vi "3axis continuous readout.vi"(6 "error in (no error)":errorcluster, 11 "VISA Gaussmeter":refnum<visa-resource-name>="GPIB1::11::INSTR") -> (4 "error out":errorcluster, 5 "VISA resource name":refnum<visa-resource-name>)   [LabVIEW 2013]
uses:
  gaussmeter channels.ctl
panel:
  in  "stop":bool
  in  "sample interval (sec)":dbl=0.1 format="%#_13g"
  out "Channel 3":dbl format="%.2f"
  in  "channel 3":T1=enum."Z"
  out "Channel 3":cluster{dbl, dbl}[](graph)
  in  "channel 2":T1=enum."Y"
  in  "channel 1":T1
  out "Channel 2":cluster{dbl, "magnetic field (T)":dbl}[](graph)
  out "Channel 1":cluster{dbl, dbl}[](graph)
  out "Channel 2":dbl format="%.2f"
  out "Channel 1":dbl format="%.2f"
  # "This .vi reads continuously \nthe values from\nthe Gaussmeter."
  # "Be aware that Hall sensors have\na stabilization time of approx. 3 sec and max. readout rate Gaussmeter: 18 rds/s"
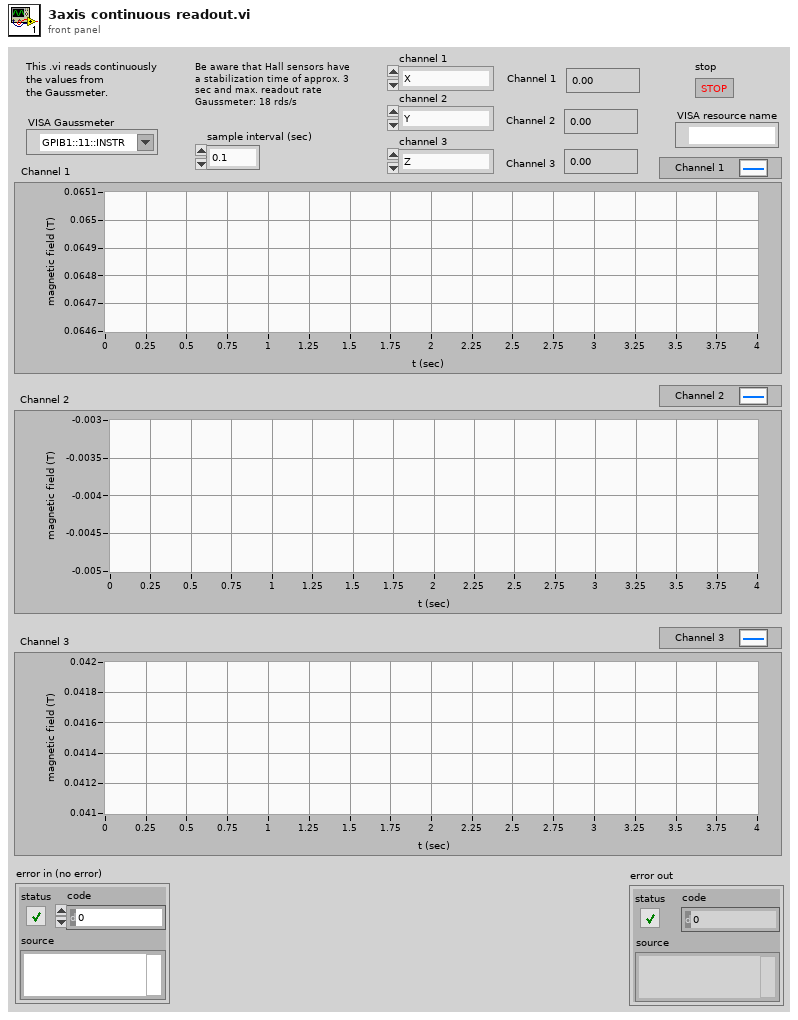
[diagram p1: front panel]
types:
  T1 = typedef "gaussmeter channels.ctl" = enum16{"X", "Y", "Z", "Vec"}
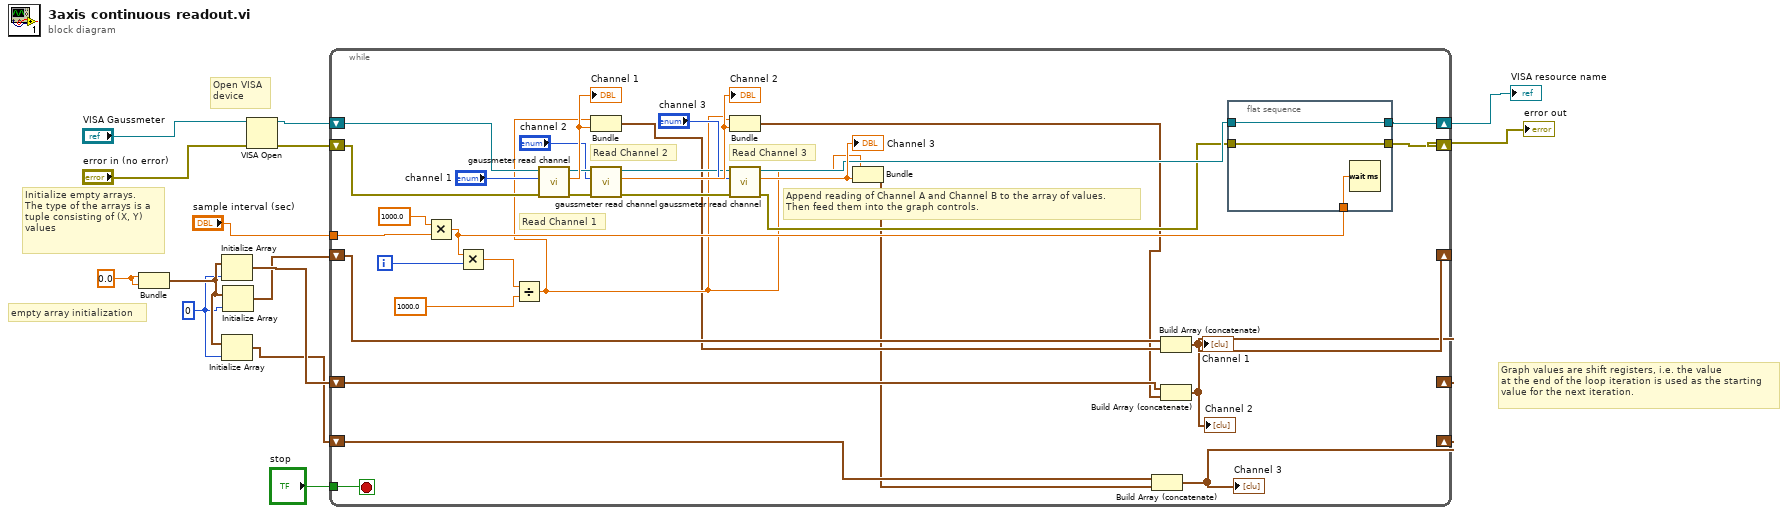
[diagram p0: block diagram]
diagram:
  w4 = 0
  w6 = 0.0
  # "empty array initialization"
  # "Graph values are shift registers, i.e. the value\nat the end of the loop iteration is used as the starting\nvalue for the next iteration."
  # "Initialize empty arrays.\nThe type of the arrays is a tuple consisting of (X, Y) values"
  # "Open VISA\ndevice"
  n1 = Bundle(w6, w6) -> (w5:cluster{dbl, dbl})  [unwired: 1 in]
  n2 = Initialize Array(w5, w4) -> (w10:cluster{dbl, dbl}[])
  n3 = Initialize Array(w5, w4) -> (w3:cluster{dbl, dbl}[])
  n4 = Initialize Array(w5, w4) -> (w9:cluster{dbl, dbl}[])
  n5 = VISA Open(error in (no error)="error in (no error)", VISA resource name="VISA Gaussmeter") -> (VISA resource name=w12:refnum<visa-resource-name>, error out=w11:errorcluster)  [unwired: 3 in]
  n6 = while {
    shift-right: [w27] -> w8
    shift-left: w11 -> [w30]
    shift-right: [w26] -> w7
    shift-left: w12 -> [w43]
    shift-right: [w47] -> _
    shift-left: w9 -> [w44]
    shift-right: [w46] -> _
    shift-left: w10 -> [w45]
    shift-right: [w42] -> _
    shift-left: w3 -> [w41]
    tunnel: "sample interval (sec)" -> [w25]
    tunnel: "stop" -> [w15]
    i -> [w23]
    stop <- w15 stop-if-true
    # "Read Channel 3"
    # "Append reading of Channel A and Channel B to the array of values.\nThen feed them into the graph controls."
    # "Read Channel 2"
    # "Read Channel 1"
    n7 = Multiply(x=1000.0, y=w25) -> (x*y=w22:dbl)
    n8 = Multiply(x=w22, y=w23) -> (x*y=w21:dbl)
    n9 = Divide(x=w21, y=1000.0) -> (x/y=w19:dbl)
    n10 = call "gaussmeter read channel.vi"("error in (no error)"=w30, "channel"="channel 1", "VISA resource name"=w43) -> ("error out"=w37:errorcluster, "magnetic field (T)"=w39:dbl, "VISA resource name 2"=w38:refnum<visa-resource-name>)  [unwired: 6 in]
    "Channel 1" <- w39
    n11 = Bundle(w19, "magnetic field (T)"=w39) -> (w18:cluster{dbl, "magnetic field (T)":dbl})  [unwired: 1 in]
    n12 = call "gaussmeter read channel.vi"("error in (no error)"=w37, "channel"="channel 2", "VISA resource name"=w38) -> ("error out"=w32:errorcluster, "magnetic field (T)"=w35:dbl, "VISA resource name 2"=w33:refnum<visa-resource-name>)  [unwired: 6 in]
    "Channel 2" <- w35
    n13 = Bundle(w19, "magnetic field (T)"=w35) -> (w17:cluster{dbl, "magnetic field (T)":dbl})  [unwired: 1 in]
    n14 = call "gaussmeter read channel.vi"("error in (no error)"=w32, "channel"="channel 3", "VISA resource name"=w33) -> ("error out"=w28:errorcluster, "magnetic field (T)"=w31:dbl, "VISA resource name 2"=w29:refnum<visa-resource-name>)  [unwired: 6 in]
    "Channel 3" <- w31
    n15 = Bundle(w19, "magnetic field (T)"=w31) -> (w16:cluster{dbl, "magnetic field (T)":dbl})  [unwired: 1 in]
    n16 = Build Array (concatenate)(w41, w16) -> (w42:cluster{dbl, "magnetic field (T)":dbl}[])
    "Channel 3" <- w42
    n17 = Build Array (concatenate)(w44, w18) -> (w47:cluster{dbl, "magnetic field (T)":dbl}[])
    "Channel 1" <- w47
    n18 = Build Array (concatenate)(w45, w17) -> (w46:cluster{dbl, "magnetic field (T)":dbl}[])
    "Channel 2" <- w46
    n19 = flat-sequence {
      tunnel: w29 -> [w49]
      tunnel: w28 -> [w50]
      tunnel: [w50] -> w27
      tunnel: [w49] -> w26
      tunnel: w22 -> [w48]
      frame #0 {
        n20 = Wait (ms)(milliseconds to wait=w48) -> ()  [unwired: 1 out]
      }
    }
  }
  "error out" <- w8
  "VISA resource name" <- w7
